vi "BGA244_meas.vi"(8 "error in":errorcluster, 11 "VISA in":refnum<visa-resource-name>) -> (0 "error out":errorcluster, 1 "ratio2":dbl, 2 "ratio1":dbl, 3 "VISA out":refnum<visa-resource-name>, 4 "status":bool)   [LabVIEW 2019]
uses:
  <vilib>/Instr/_visa.llb/VISA Flush IO Buffer Mask.ctl
panel:
  out "string 2":string
  out "string 1":string
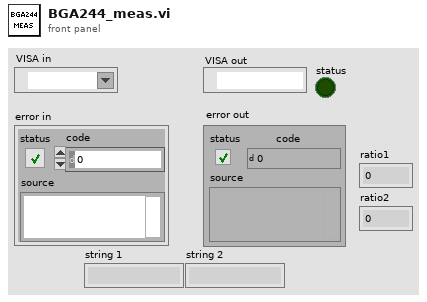
[diagram p1: front panel]
types:
  T1 = typedef "VISA Flush IO Buffer Mask.ctl" = u16
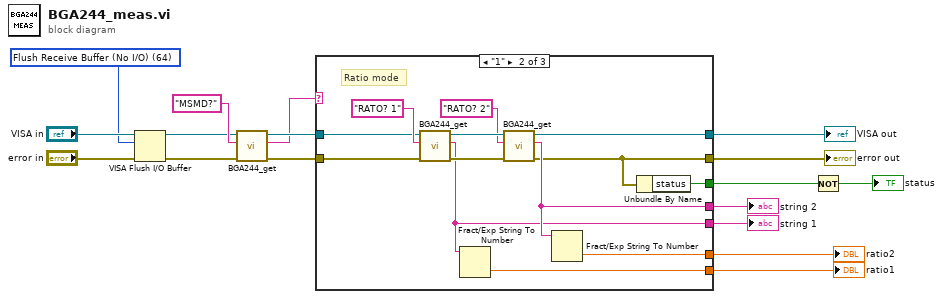
[diagram p0: block diagram]
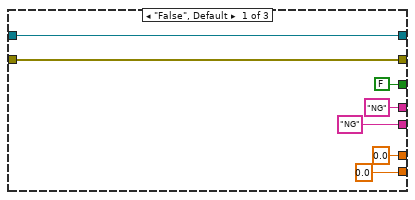
[diagram p2: hidden frame]
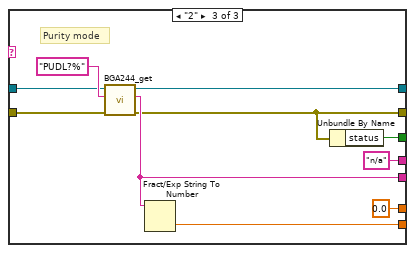
[diagram p3: hidden frame]
diagram:
  w1 = T1 64 items=["Flush Receive Buffer"=16, "Write Transmit Buffer to Device"=32, "Flush Receive Buffer (No I/O)"=64, "Flush Transmit Buffer"=128] ("Mask")
  n1 = VISA Flush I/O Buffer(VISA resource name="VISA in", mask (16)=w1, error in (no error)="error in") -> (VISA resource name out=w4:refnum<visa-resource-name>, error out=w2:errorcluster)
  n2 = call "BGA244_get.vi"("error in"=w2, "string in"="MSMD?", "VISA in"=w4) -> ("error out"=w14:errorcluster, "string out"=w11:string, "VISA out"=w13:refnum<visa-resource-name>)  [unwired: 6 in]
  n3 = case shown="\"1\"" w11 {
    tunnel: [w24 w35 w44] -> w17
    tunnel: [w23 w25 w38] -> w16
    tunnel: w14 -> [w23 w32 w45]
    tunnel: w13 -> [w24 w31 w46]
    tunnel: [0.0 w30 0.0] -> w10
    tunnel: [0.0 w29 w41] -> w9
    tunnel: ["NG" ("string out") w28 "n/a" ("string out")] -> w8
    tunnel: ["NG" ("string out") w27 w43] -> w7
    tunnel: [FALSE ("status") w26 w39] -> w6
    frame "False", Default {
    }
    frame "1" {
      # "Ratio mode"
      n4 = call "BGA244_get.vi"("error in"=w32, "string in"="RATO? 1" ("string"), "VISA in"=w31) -> ("error out"=w34:errorcluster, "string out"=w27:string, "VISA out"=w36:refnum<visa-resource-name>)  [unwired: 6 in]
      n5 = Fract/Exp String To Number(string=w27) -> (number=w29:dbl)  [unwired: 3 in, 1 out]
      n6 = call "BGA244_get.vi"("error in"=w34, "string in"="RATO? 2" ("string"), "VISA in"=w36) -> ("error out"=w25:errorcluster, "string out"=w28:string, "VISA out"=w35:refnum<visa-resource-name>)  [unwired: 6 in]
      n7 = Fract/Exp String To Number(string=w28) -> (number=w30:dbl)  [unwired: 3 in, 1 out]
      n8 = Unbundle By Name(w25) -> ("status"=w26:bool)
    }
    frame "2" {
      # "Purity mode"
      n9 = call "BGA244_get.vi"("error in"=w45, "string in"="PUDL?%" ("string"), "VISA in"=w46) -> ("error out"=w38:errorcluster, "string out"=w43:string, "VISA out"=w44:refnum<visa-resource-name>)  [unwired: 6 in]
      n10 = Fract/Exp String To Number(string=w43) -> (number=w41:dbl)  [unwired: 3 in, 1 out]
      n11 = Unbundle By Name(w38) -> ("status"=w39:bool)
    }
  }
  "VISA out" <- w17
  "error out" <- w16
  "ratio1" <- w9
  "ratio2" <- w10
  "string 2" <- w8
  "string 1" <- w7
  n12 = Not(x=w6) -> (.not. x?=→"status":bool)
